vi "mcl_query_positions.vi"(8 "error in (no error)":errorcluster, 11 "thorlabs_panel in":refnum<class "mcl_panel.lvclass">) -> (0 "error out":errorcluster, 3 "thorlabs_panel out":refnum<class "mcl_panel.lvclass">)   [LabVIEW 2015, in "mcl_panel.lvclass"]
uses:
  mcl_panel.lvclass
  mcl_piezo_class/mcl_piezo.lvclass
  mcl_panel.lvclass/mcl_panel.ctl
  UI/panel_class/panel.lvclass
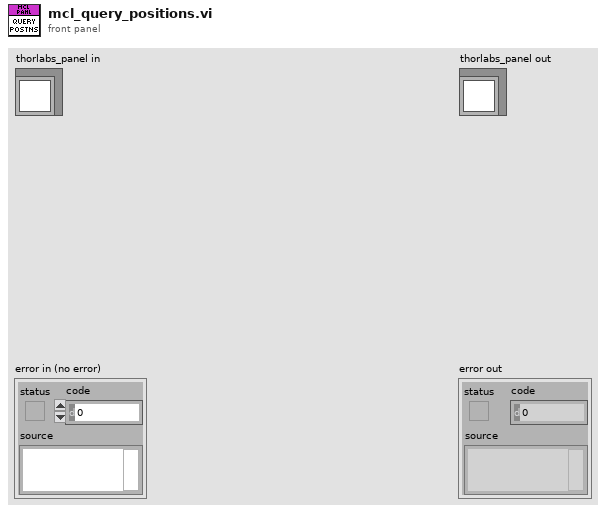
[diagram p1: front panel]
types:
  T1 = typedef "thorlabs_events.ctl" = cluster{"mcl_status":refnum<user-event>, "piezo_positions":refnum<user-event>}
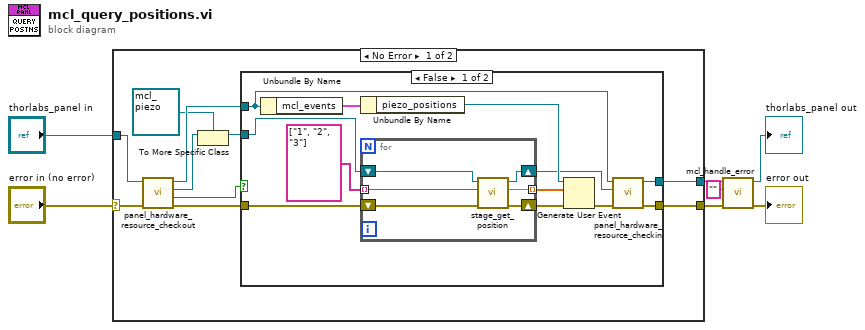
[diagram p0: block diagram]
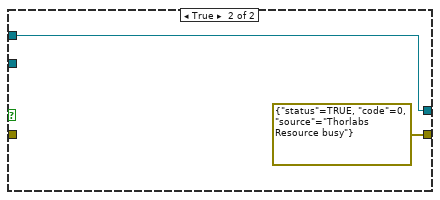
[diagram p2: hidden frame]
diagram:
  n1 = case shown="No Error" "error in (no error)" {
    selector: "error in (no error)" -> [w16 w39]
    tunnel: [w9 w39] -> w2
    tunnel: "thorlabs_panel in" -> [w17 w38]
    tunnel: [w10 w38] -> w4
    frame No Error {
      n2 = call "panel_hardware_resource_checkout.vi"("error in (no error)"=w16, "panel in"=w17) -> ("error out"=w13:errorcluster, "timed out?"=w12:bool, "hardware.lvclass"=w15:refnum<class "hardware.lvclass">, "panel out"=w11:refnum<class "mcl_panel.lvclass">)  [unwired: 6 in]
      n3 = To More Specific Class(target class=refnum<class "mcl_piezo.lvclass"> refnum ("mcl_piezo.lvclass"), reference=w15) -> (specific class reference=w14:refnum<class "mcl_piezo.lvclass">)  [unwired: 1 in, 1 out]
      n4 = case shown="False" w12 {
        tunnel: w14 -> [w27 _]
        tunnel: w13 -> [w26 _]
        tunnel: w11 -> [w25 w36]
        tunnel: [w29 w36] -> w10
        tunnel: [w28 errorcluster {"status"=TRUE, "code"=0, "source"="Thorlabs Resource busy"} ("error out")] -> w9
        frame False {
          n5 = Unbundle By Name(w25) -> ("mcl_events"=w24:T1)
          n6 = Unbundle By Name(w24) -> ("piezo_positions"=w23:refnum<user-event>)
          n7 = for {
            shift-right: [w31] -> w21
            shift-left: w26 -> [w32]
            shift-right: [w34] -> w18
            shift-left: w27 -> [w35]
            tunnel: string[] ["1", "2", "3"] -> [w30] mode=indexing
            tunnel: [w33] -> w19 mode=indexing
            n8 = call-dynamic "stage_get_position.vi"("error in (no error)"=w32, "Stage Name"=w30, "mcl_piezo in"=w35) -> ("error out"=w31:errorcluster, "Position"=w33:dbl, "mcl_piezo out"=w34:refnum<class "mcl_piezo.lvclass">)  [unwired: 6 in]
          }
          n9 = Generate User Event(user event=w23, event data cluster=w19, error in=w21) -> (error out=w22:errorcluster)  [unwired: 1 in, 1 out]
          n10 = call "panel_hardware_resource_checkin.vi"("error in (no error)"=w22, "hardware.lvclass"=w18, "panel in"=w25) -> ("error out"=w28:errorcluster, "panel out"=w29:refnum<class "mcl_panel.lvclass">)  [unwired: 7 in]
        }
        frame True {
        }
      }
    }
    frame Error {
    }
  }
  n11 = call "mcl_handle_error.vi"("error in (no error)"=w2, "No Error String"="", "thorlabs_panel in"=w4) -> ("error out"=→"error out":errorcluster, "thorlabs_panel out"=→"thorlabs_panel out":refnum<class "mcl_panel.lvclass">)  [unwired: 7 in]
